vi "Sender.vi"() -> ()   [LabVIEW 2019]
uses:
  <vilib>/vision/NI_Vision_Development_Module.lvlib
panel:
  out "Status":string
  in  "stop":bool
  in  "port":u16=3015
  out "Image":T1(plugin-control)
  # "First start This VI,\nthen start receiver"
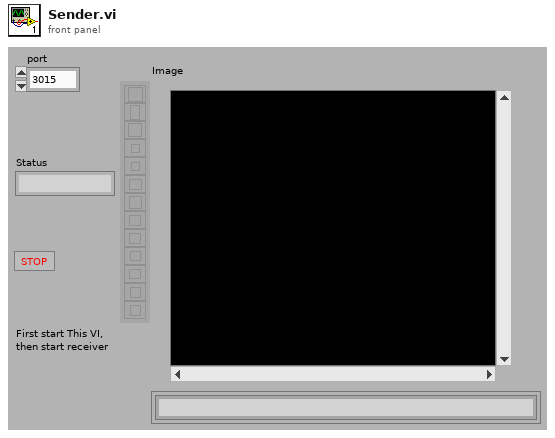
[diagram p1: front panel]
types:
  T1 = typedef "IMAQ Image.ctl" = refnum<image>
  T2 = typedef "Image Type" = u32
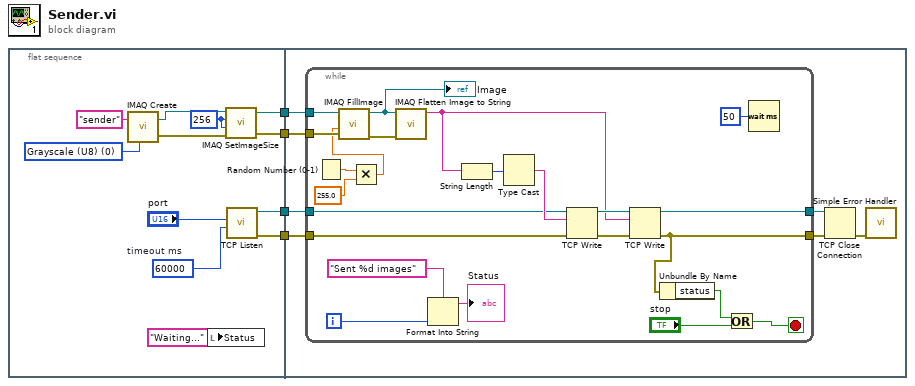
[diagram p0: block diagram]
diagram:
  n1 = flat-sequence {
    tunnel: [w7] -> w4
    tunnel: [w6] -> w3
    tunnel: [w9] -> w2
    tunnel: [w8] -> w1
    tunnel: w4 -> [w23]
    tunnel: w3 -> [w22]
    tunnel: w2 -> [w21]
    tunnel: w1 -> [w20]
    frame #0 {
      w16 = 256 ("X Resolution")
      w12 = 60000  # timeout ms
      w11 = T2 0 items=["Grayscale (U8)", "Grayscale (I16)", "Grayscale (SGL)", "Complex (CSG)", "RGB (U32)", "HSL (U32)", "RGB (U64)"] ("Image Type")
      n2 = call "IMAQ Create"("Image Name"="sender", "Image Type"=w11) -> ("New Image"=w14:T1, "error out"=w15:errorcluster)  [unwired: 3 in]
      n3 = local write "Status"("Waiting..." ("Status")) -> ()
      n4 = call "IMAQ SetImageSize"("error in (no error)"=w15, "Y Resolution"=w16, "X Resolution"=w16, "Image"=w14) -> ("error out"=w8:errorcluster, "Image Out"=w9:T1)  [unwired: 1 in]
      n5 = call <vilib>:"TCP Listen.vi"("timeout ms (wait forever: -1)"=w12, "port"="port") -> ("error out"=w6:errorcluster, "connection ID"=w7:refnum<k5>)  [unwired: 5 in, 3 out]
    }
    frame #1 {
      n6 = while {
        tunnel: w23 -> [w44]
        tunnel: w22 -> [w43]
        tunnel: w21 -> [w36]
        tunnel: w20 -> [w35]
        tunnel: [w26] -> w19
        tunnel: [w25] -> w17
        i -> [w29]
        stop <- w38 stop-if-true
        n7 = Random Number (0-1)() -> (number: 0 to 1=w33:dbl)
        n8 = Multiply(x=w33, y=255.0) -> (x*y=w31:dbl)
        n9 = call "IMAQ FillImage"("error in (no error)"=w35, "Pixel Value (U8, U16, I16, Float)"=w31, "Image"=w36) -> ("error out"=w34:errorcluster, "Image Out"=w27:T1)  [unwired: 7 in]
        "Image" <- w27
        n10 = call "IMAQ Flatten Image to String"("error in (no error)"=w34, "Image"=w27) -> ("Data String"=w40:string)  [unwired: 8 in, 1 out]
        n11 = Format Into String(format string="Sent %d images", w29) -> (resulting string=→"Status":string)  [unwired: 2 in, 1 out]
        n12 = String Length(string=w40) -> (length=w46:i32)
        n13 = Type Cast(x=w46) -> (*(type *) &x=w45:string)  [unwired: 1 in]
        n14 = TCP Write(connection ID=w44, data in=w45, error in (no error)=w43) -> (connection ID out=w42:refnum<k5>, error out=w41:errorcluster)  [unwired: 1 in, 1 out]
        n15 = TCP Write(connection ID=w42, data in=w40, error in (no error)=w41) -> (connection ID out=w25:refnum<k5>, error out=w26:errorcluster)  [unwired: 1 in, 1 out]
        n16 = Unbundle By Name(w26) -> ("status"=w37:bool)
        n17 = Or(x=w37, y="stop") -> (x .or. y?=w38:bool)
        n18 = Wait (ms)(milliseconds to wait=u32 50) -> ()  [unwired: 1 out]
      }
      n19 = TCP Close Connection(connection ID=w17, error in (no error)=w19) -> (error out=w18:errorcluster)  [unwired: 1 in, 1 out]
      n20 = call <vilib>:"Simple Error Handler.vi"("error in (no error)"=w18) -> ()  [unwired: 4 in, 5 out]
    }
  }
